vi "GOLPI simple testing.vi"() -> ()   [LabVIEW 2020, in "GOLPI library.lvlib"]
uses:
  GOLPI library.lvlib
  Get Variable - polymorph parts/Get String.vi
  Get Variable - polymorph parts/Get Double.vi
  Get Variable - polymorph parts/Get Double Complex.vi
  Get Variable - polymorph parts/Get 1D Array Double.vi
  Get Variable - polymorph parts/Get 1D Array String.vi
  Get Variable - polymorph parts/Get 1D Array Double Complex.vi
  Get Variable - polymorph parts/Get 2D Array Double.vi
  Get Variable - polymorph parts/Get 2D Array Double Complex.vi
panel:
  in  "Variable Pipe Mode?":bool
  in  "wait for exit\n(press this again to exit)":bool=TRUE
  in  "Bitstream mode?":bool
  in  "hide debug console":bool
  in  "data type array 5":cdb[][](array[numeric])
  in  "data type array 4":dbl[][](array[numeric])
  in  "use temporary file?":bool
  in  "data type array 3":cdb[](array[numeric])
  in  "data type array 2":string[](array[string])
  in  "data type 4":cdb
  in  "data type 3":dbl
  in  "Get variable":T1(tab)=enum."vector reals"
  out "s":string
  out "r":dbl format="%.2f"
  out "c":cdb format="%.2f"
  out "vs length":i32
  out "vs":string[](array[string])
  out "vr":dbl[](array[numeric])
  out "vr length":i32
  out "vc length":i32
  out "vc":cdb[](array[numeric])
  out "mr":dbl[][](array[numeric]) format="%.2f"
  out "mr sizes":i32[](array[numeric])
  out "mc sizes":i32[](array[numeric])
  out "mc":cdb[][](array[numeric]) format="%.2f"
  in  "data type array":dbl[](array[numeric])
  in  "data type":string
  in  "variable name":string="x"
  in  "command":string="x=[1 2 3]\ndisp('OK')"
  out "GNU Octave version":string
  out "exit code":i32
  out "error out":errorcluster
  out "read buffer":string
  in  "Octave binary directory":path=path "C:/Octave/Octave-4.2.2/bin/octave-cli.exe"
  in  "Working directory":path=path "C:/work"
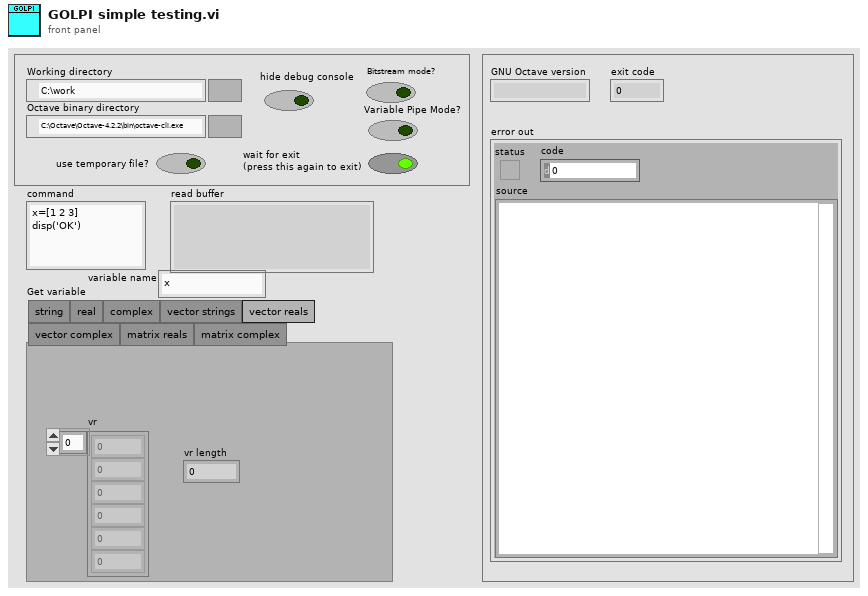
[diagram p1: front panel]
types:
  T1 = enum32{"string", "real", "complex", "vector strings", "vector reals", "vector complex", "matrix reals", "matrix complex"}
  T2 = typedef "GOLPI library.lvlib/GOLPI reference Type Def.ctl" = cluster{"pipe handle":T3, "fast read timeout [ms]":u32, "fast read settle time [ms]":u32, "fast read to multiple [ms]":u32, "max elements per input line":u32, "slow read timeout [ms]":u32, "stdin double format specifier":string, "max elements per stdout output column":u32, "console mode bitstream":bool, "bitstream first read timeout [ms]":u32, "bitstream read timeout [ms]":u32, "struct transfer possible":bool, "matlab mode":bool, "var pipe write timeout [ms]":u32, "variable pipe mode":bool, "variable pipe buffer size [Bytes]":u32, "variable pipe block size [Bytes]":u32}
  T3 = typedef "LV Process library.lvlib/Pipe Handle.ctl" = cluster{"lv_proc.dll file path":path, "process instance handle":u32[], "debug mode":bool, "debug data":cluster{"time":timestamp, "stdin":bool, "data":string}[]}
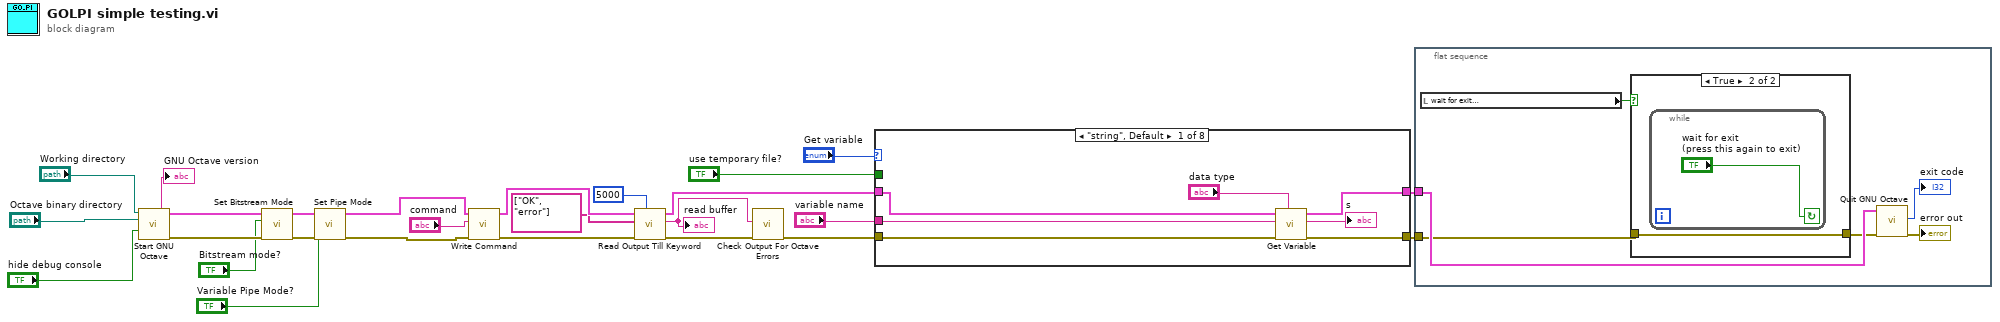
[diagram p0: block diagram]
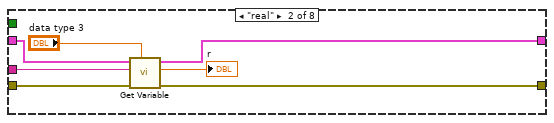
[diagram p3: hidden frame]
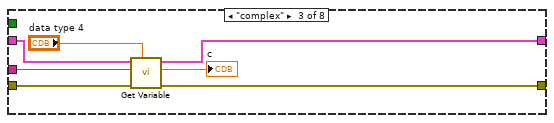
[diagram p4: hidden frame]
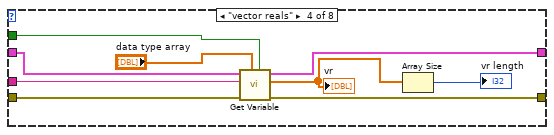
[diagram p5: hidden frame]
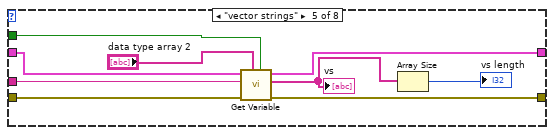
[diagram p6: hidden frame]
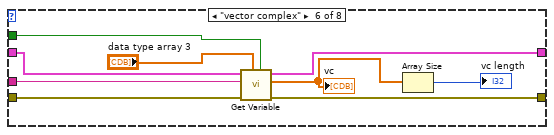
[diagram p7: hidden frame]
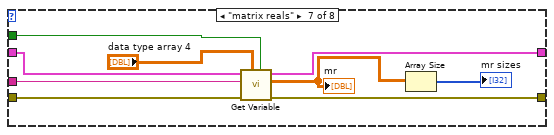
[diagram p8: hidden frame]
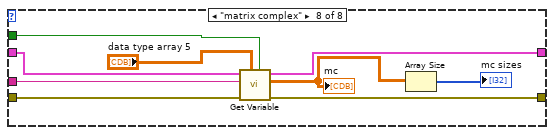
[diagram p9: hidden frame]
diagram:
  n1 = call "Start GNU Octave.vi"("working dir (user home)"="Working directory", "octave binary file or dir (autofind)"="Octave binary directory", "hide debug console (T)"="hide debug console") -> ("GNU Octave version"=→"GNU Octave version":string, "GOLPI ref. out"=w8:T2, "error out"=w9:errorcluster)  [unwired: 9 in, 1 out]
  n2 = call "Set Bitstream Mode.vi"("error in"=w9, "Bitstream mode (F)"="Bitstream mode?", "GOLPI ref. in"=w8) -> ("error out"=w5:errorcluster, "GOLPI ref. out"=w4:T2)  [unwired: 7 in]
  n3 = call "Set Pipe Mode.vi"("error in"=w5, "Variable Pipe Mode? (F)"="Variable Pipe Mode?", "GOLPI ref. in"=w4) -> ("error out"=w2:errorcluster, "GOLPI ref. out"=w3:T2)  [unwired: 7 in]
  n4 = call "Write Command.vi"("error in"=w2, "command"="command", "GOLPI ref. in"=w3) -> ("error out"=w23:errorcluster, "GOLPI ref. out"=w24:T2)  [unwired: 7 in]
  n5 = call "Read Output Till Keyword.vi"("timeout [ms]"=u32 5000, "error in"=w23, "keywords"=string[] ["OK", "error"], "GOLPI ref. in"=w24) -> ("error out"=w19:errorcluster, "read buffer"=w17:string, "GOLPI ref. out"=w22:T2)  [unwired: 4 in, 1 out]
  "read buffer" <- w17
  n6 = call "Check Output For Octave Errors.vi"("error in"=w19, "read buffer"=w17) -> ("error out"=w18:errorcluster)  [unwired: 9 in]
  n7 = case shown="\"string\", Default" "Get variable" {
    tunnel: w22 -> [w32 w37 w45 w54 w62 w70 w83 w91]
    tunnel: [w29 w35 w42 w53 w59 w67 w79 w88] -> w21
    tunnel: [w30 w34 w41 w52 w60 w68 w80 w87] -> w6
    tunnel: "variable name" -> [w27 w38 w43 w55 w63 w71 w82 w89]
    tunnel: w18 -> [w31 w39 w44 w56 w61 w69 w81 w90]
    tunnel: "use temporary file?" -> [_ _ _ w49 w57 w66 w78 w86]
    frame "string", Default {
      n8 = call-poly "Get Variable.vi"("data type of variable"="data type", "error in"=w31, "variable name"=w27, "GOLPI ref. in"=w32) -> ("error out"=w30:errorcluster, "value"=→"s":string, "GOLPI ref. out"=w29:T2)  [unwired: 5 in]
    }
    frame "real" {
      n9 = call-poly "Get Variable.vi"("data type of variable"="data type 3", "error in"=w39, "variable name"=w38, "GOLPI ref. in"=w37) -> ("error out"=w34:errorcluster, "value"=→"r":dbl, "GOLPI ref. out"=w35:T2)  [unwired: 5 in]
    }
    frame "complex" {
      n10 = call-poly "Get Variable.vi"("data type of variable"="data type 4", "error in"=w44, "variable name"=w43, "GOLPI ref. in"=w45) -> ("error out"=w41:errorcluster, "value"=→"c":cdb, "GOLPI ref. out"=w42:T2)  [unwired: 5 in]
    }
    frame "vector reals" {
      n11 = call-poly "Get Variable.vi"("use temporary file? (F)"=w49, "data type of variable"="data type array", "error in"=w56, "variable name"=w55, "GOLPI ref. in"=w54) -> ("error out"=w52:errorcluster, "value"=w48:dbl[], "GOLPI ref. out"=w53:T2)  [unwired: 4 in]
      "vr" <- w48
      n12 = Array Size(array=w48) -> (size(s)=→"vr length":i32)
    }
    frame "vector strings" {
      n13 = call-poly "Get Variable.vi"("use temporary file? (F)"=w57, "data type of variable"="data type array 2", "error in"=w61, "variable name"=w63, "GOLPI ref. in"=w62) -> ("error out"=w60:errorcluster, "value"=w58:string[], "GOLPI ref. out"=w59:T2)  [unwired: 4 in]
      "vs" <- w58
      n14 = Array Size(array=w58) -> (size(s)=→"vs length":i32)
    }
    frame "vector complex" {
      n15 = call-poly "Get Variable.vi"("use temporary file? (F)"=w66, "data type of variable"="data type array 3", "error in"=w69, "variable name"=w71, "GOLPI ref. in"=w70) -> ("error out"=w68:errorcluster, "value"=w72:cdb[], "GOLPI ref. out"=w67:T2)  [unwired: 4 in]
      "vc" <- w72
      n16 = Array Size(array=w72) -> (size(s)=→"vc length":i32)
    }
    frame "matrix reals" {
      n17 = call-poly "Get Variable.vi"("use temporary file? (F)"=w78, "data type of variable"="data type array 4", "error in"=w81, "variable name"=w82, "GOLPI ref. in"=w83) -> ("error out"=w80:errorcluster, "value"=w75:dbl[][], "GOLPI ref. out"=w79:T2)  [unwired: 4 in]
      "mr" <- w75
      n18 = Array Size(array=w75) -> (size(s)=→"mr sizes":i32[])
    }
    frame "matrix complex" {
      n19 = call-poly "Get Variable.vi"("use temporary file? (F)"=w86, "data type of variable"="data type array 5", "error in"=w90, "variable name"=w89, "GOLPI ref. in"=w91) -> ("error out"=w87:errorcluster, "value"=w84:cdb[][], "GOLPI ref. out"=w88:T2)  [unwired: 4 in]
      "mc" <- w84
      n20 = Array Size(array=w84) -> (size(s)=→"mc sizes":i32[])
    }
  }
  n21 = flat-sequence {
    tunnel: w21 -> [w96]
    tunnel: w6 -> [w94]
    frame #0 {
      n22 = local read "wait for exit\n(press this again to exit)"() -> (w95:bool)
      n23 = case shown="True" w95 {
        tunnel: [w99 w100] -> w93
        tunnel: w94 -> [w99 w100]
        frame False {
        }
        frame True {
          n24 = while {
            stop <- "wait for exit\n(press this again to exit)" continue-if-true
          }
        }
      }
      n25 = call "Quit GNU Octave.vi"("error in"=w93, "GOLPI ref. in"=w96) -> ("error out"=→"error out":errorcluster, "exit code"=→"exit code":i32)  [unwired: 8 in]
    }
  }
